vi "Get Generic Property (Core).vi"(0 "SLSC Interface in":refnum<class "SLSC Interface.lvclass">, 1 "property type":T1, 5 "resources":string, 7 "property":refnum<k21>, 11 "error in (no error)":errorcluster) -> (4 "SLSC Interface out":refnum<class "SLSC Interface.lvclass">, 10 "property value":variant, 15 "error out":errorcluster)   [LabVIEW 2016, in "SLSC Interfaces.lvlib" / "SLSC Interface.lvclass"]
uses:
  SLSC Interface.lvclass
  Property Type.ctl
  SLSC Interface.lvclass/SLSC Interface.ctl
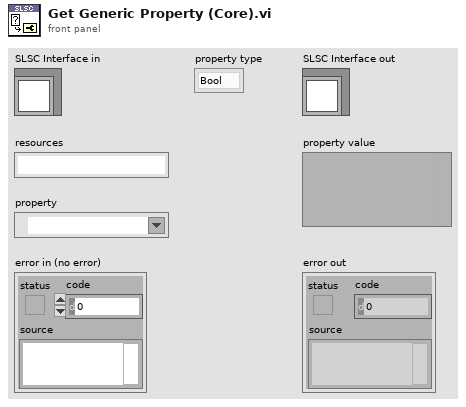
[diagram p1: front panel]
types:
  T1 = typedef "SLSC Interfaces.lvlib/SLSC Interface.lvclass/property type.ctl" = enum16{"Bool", "DBL", "I32", "I64", "String", "U32", "U64", "1D Bool", "1D DBL", "1D I32", "1D I64", "1D String", "1D U32", "1D U64"}
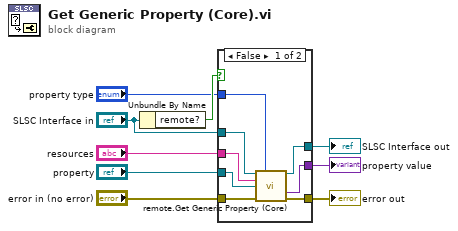
[diagram p0: block diagram]
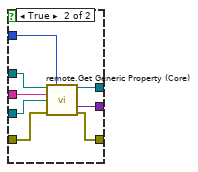
[diagram p2: hidden frame]
diagram:
  n1 = Unbundle By Name("SLSC Interface in") -> ("remote?"=w9:bool)
  n2 = case shown="False" w9 {
    tunnel: "SLSC Interface in" -> [w16 w25]
    tunnel: "resources" -> [w14 w24]
    tunnel: "property" -> [w13 w23]
    tunnel: "error in (no error)" -> [w12 w22]
    tunnel: [w17 w21] -> w4
    tunnel: [w10 w20] -> w3
    tunnel: [w11 w19] -> w2
    tunnel: "property type" -> [w15 w18]
    frame False {
      n3 = call "remote.Get Generic Property (Core).vi"("SLSC Remote in"=w16, "property type"=w15, "resources"=w14, "property"=w13, "error in (no error)"=w12) -> ("SLSC Remote out"=w17:refnum<class "SLSC Interface.lvclass">, "property value"=w10:variant, "error out"=w11:errorcluster)  [unwired: 8 in]
    }
    frame True {
      n4 = call "remote.Get Generic Property (Core).vi"("SLSC Remote in"=w25, "property type"=w18, "resources"=w24, "property"=w23, "error in (no error)"=w22) -> ("SLSC Remote out"=w21:refnum<class "SLSC Interface.lvclass">, "property value"=w20:variant, "error out"=w19:errorcluster)  [unwired: 8 in]
    }
  }
  "error out" <- w2
  "SLSC Interface out" <- w4
  "property value" <- w3
